vi "Potting Data - TBM HDI.vi"(10 "TBM-HDI Selection":T6, 11 "TBM-HDI Data":T2) -> (3 "Potting Lines":T1[](array[typedef]))   [LabVIEW 2011]
uses:
  Shared Components/Utils/Type Definitions/Multi-Fiducial Image.ctl
  Shared Components/Vec3d Class/Vec3d Class.lvclass
  Shared Components/Utils/Type Definitions/Physical Image.ctl
  <vilib>/vision/Image Controls.llb/IMAQ Image.ctl
  Shared Components/Utils/Type Definitions/Fiducial with Source.ctl
  Shared Components/Utils/Type Definitions/3d Line.ctl
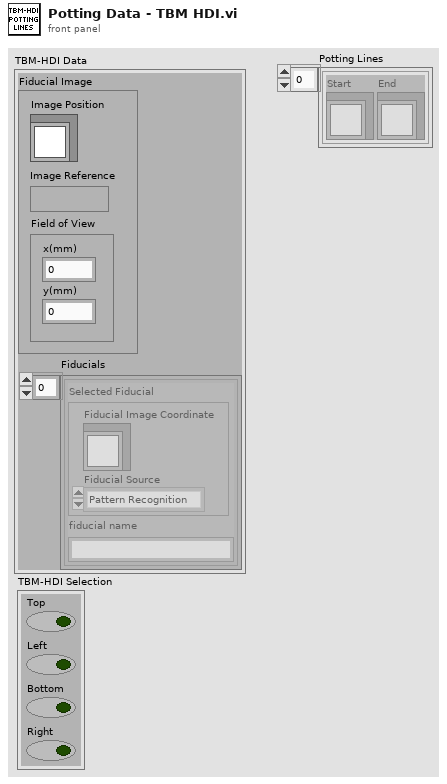
[diagram p1: front panel]
types:
  T1 = typedef "3d Line.ctl" = cluster{"Start":refnum<class "Vec3d Class.lvclass">, "End":refnum<class "Vec3d Class.lvclass">}
  T2 = typedef "Multi-Fiducial Image.ctl" = cluster{"Fiducial Image":T3, "Fiducials":cluster{"Selected Fiducial":T5, "fiducial name":string}[]}
  T3 = typedef "Physical Image.ctl" = cluster{"Image Position":refnum<class "Vec3d Class.lvclass">, "Image Reference":T4, "Field of View":cluster{"x(mm)":dbl, "y(mm)":dbl}}
  T4 = typedef "IMAQ Image.ctl" = refnum<image>
  T5 = typedef "Fiducial with Source.ctl" = cluster{"Fiducial Image Coordinate":refnum<class "Vec3d Class.lvclass">, "Fiducial Source":enum16{"Pattern Recognition", "User", "Error", "Default"}}
  T6 = cluster{"Top":bool, "Left":bool, "Bottom":bool, "Right":bool}
  T7 = cluster{"Selected Fiducial":T5, "fiducial name":string}[]
  T8 = cluster{"Selected Fiducial":T5, "fiducial name":string}
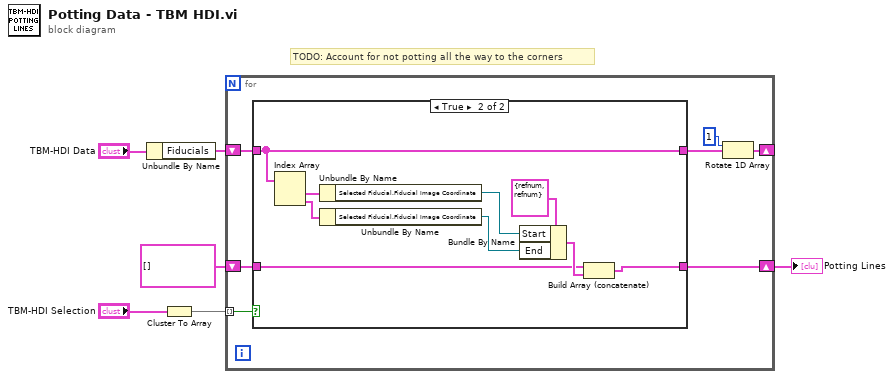
[diagram p0: block diagram]
diagram:
  # "TODO: Account for not potting all the way to the corners"
  n1 = Unbundle By Name("TBM-HDI Data") -> ("Fiducials"=w3:T7)
  n2 = Cluster To Array(cluster="TBM-HDI Selection") -> (array=w4:bool[])
  n3 = for {
    tunnel: w4 -> [w13] mode=indexing
    shift-right: [w7] -> _
    shift-left: w3 -> [w12]
    shift-right: [w10] -> w1
    shift-left: T1[] [] -> [w11]
    n4 = case shown="True" w13 {
      tunnel: w12 -> [w14 w24]
      tunnel: [w14 w24] -> w8
      tunnel: w11 -> [w15 w17]
      tunnel: [w15 w16] -> w10
      frame False {
      }
      frame True {
        n5 = Index Array(array=w24) -> (element #1=w22:T8, element #2=w23:T8)  [unwired: 2 in]
        n6 = Unbundle By Name(w22) -> ("Selected Fiducial.Fiducial Image Coordinate"=w20:refnum<class "Vec3d Class.lvclass">)
        n7 = Unbundle By Name(w23) -> ("Selected Fiducial.Fiducial Image Coordinate"=w19:refnum<class "Vec3d Class.lvclass">)
        n8 = Bundle By Name(cluster=T1 {"Start"=refnum, "End"=refnum} ("3D Line"), "Start"=w20, "End"=w19) -> (w18:T1)
        n9 = Build Array (concatenate)(w17, w18) -> (w16:T1[])
      }
    }
    n10 = Rotate 1D Array(1:w8, 2:1 ("n")) -> (0:w7:T7)
  }
  "Potting Lines" <- w1
